vi "my_solution.vi"() -> ()   [LabVIEW 2013]
doc: "This example performs writes and reads on a serial port, as directed by the user. You can press the Write and Read buttons, and change the Read Count, while the example is running.\n\nThe parameters set for the serial port must match the parameters of the connected instrument or device. In this example, the Read Count parameter specifies the number of bytes that the serial port reads. If there were more bytes at the port than the specified number, those bytes would not be read. If there were less bytes at the port than the specified number, you would receive a timeout error.\n\nThis example expands upon the flow control options for XON and XOFF, allowing the user to choose those control characters. Also, the user can enable or disable a termination character. Some devices require a termination character in order to identify the end of command strings. Some devices send a termination character to signify the end of data to be read. This example shows how you can end the Read operation once a termination character is detected in the buffer and/or append a termination character at the end of the Write data."
uses:
  Program Files/National Instruments/LabVIEW 2013/examples/Instrument IO/Serial/support/Serial - Settings.ctl
  <vilib>/Instr/_visa.llb/VISA Configure Serial Port (Instr).vi
panel:
  out "device 4":bool
  out "device 3":bool
  out "Waveform Chart 9":T1(graph)
  out "Waveform Chart 8":T1(graph)
  out "Waveform Chart 7":T1(graph)
  out "unit type 3":dbl
  out "time3":dbl
  in  "Write 4":bool
  in  "Write 3":bool
  out "goniometer":u8(knob) scale=0.0..255.0
  out "unit type":dbl
  out "Waveform Chart 6":T1(graph)
  out "Waveform Chart 5":T1(graph)
  out "Waveform Chart 4":T1(graph)
  out "unit type 2":dbl
  out "time 2":dbl
  out "device 2":bool
  out "device 1":bool
  out "time":dbl
  in  "Write 2":bool
  out "Waveform Chart 3":T1(graph)
  out "Waveform Chart 2":T1(graph)
  out "Waveform Chart":T1(graph)
  in  "Stop":bool
  in  "Command":string="*IDN?"
  in  "Write":bool
  in  "Serial Settings":T2={"baud rate"=115200, "data bits"=8, "parity"=enum."None", "stop bits"=10, "flow control"=0} {"flow control" items=["None"=0, "XON/XOFF"=1, "RTS/CTS"=2, "DTR/DSR"=4]; "stop bits" items=["1.0"=10, "1.5"=15, "2.0"=20]; "data bits" min=5 max=8 step=1; "baud rate" items=["75"=75, "110"=110, "134"=134, "150"=150, "300"=300, "600"=600, "1200"=1200, "1800"=1800, "2400"=2400, "4800"=4800, "7200"=7200, "9600"=9600, "14400"=14400, "19200"=19200, "28800"=28800, "38400"=38400, "56000"=56000, "57600"=57600, "115200"=115200, "128000"=128000, "230400"=230400]}
  in  "VISA resource name":refnum<visa-resource-name>="COM4"
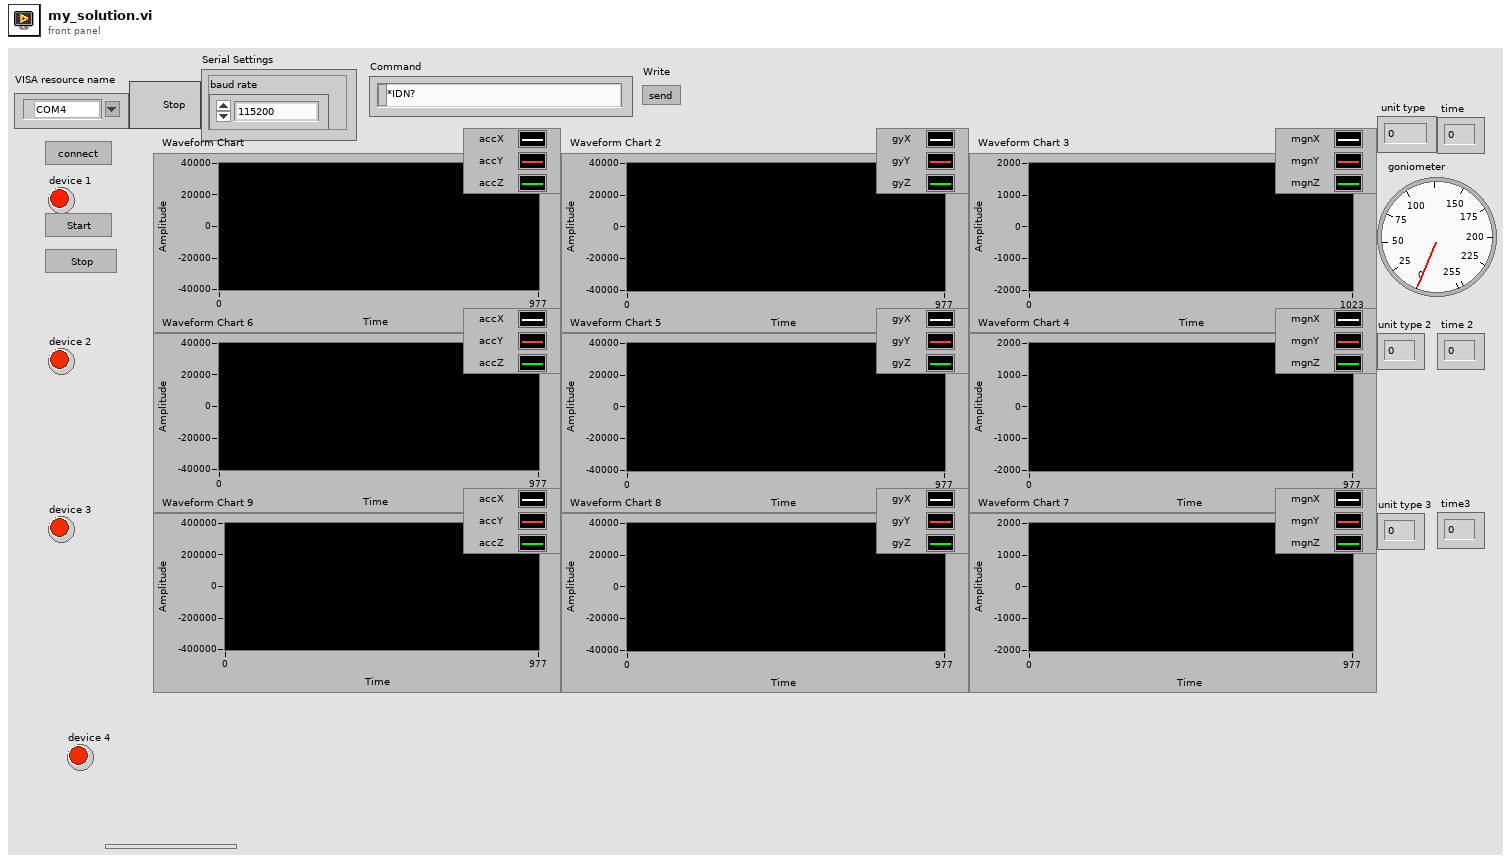
[diagram p1: front panel]
types:
  T1 = cluster{"Numeric Control":dbl, "Numeric Control":dbl, "Numeric Control":dbl}
  T2 = typedef "Serial - Settings.ctl" = cluster{"baud rate":u32, "data bits":u16, "parity":enum16{"None", "Odd", "Even", "Mark", "Space"}, "stop bits":u16, "flow control":u16}
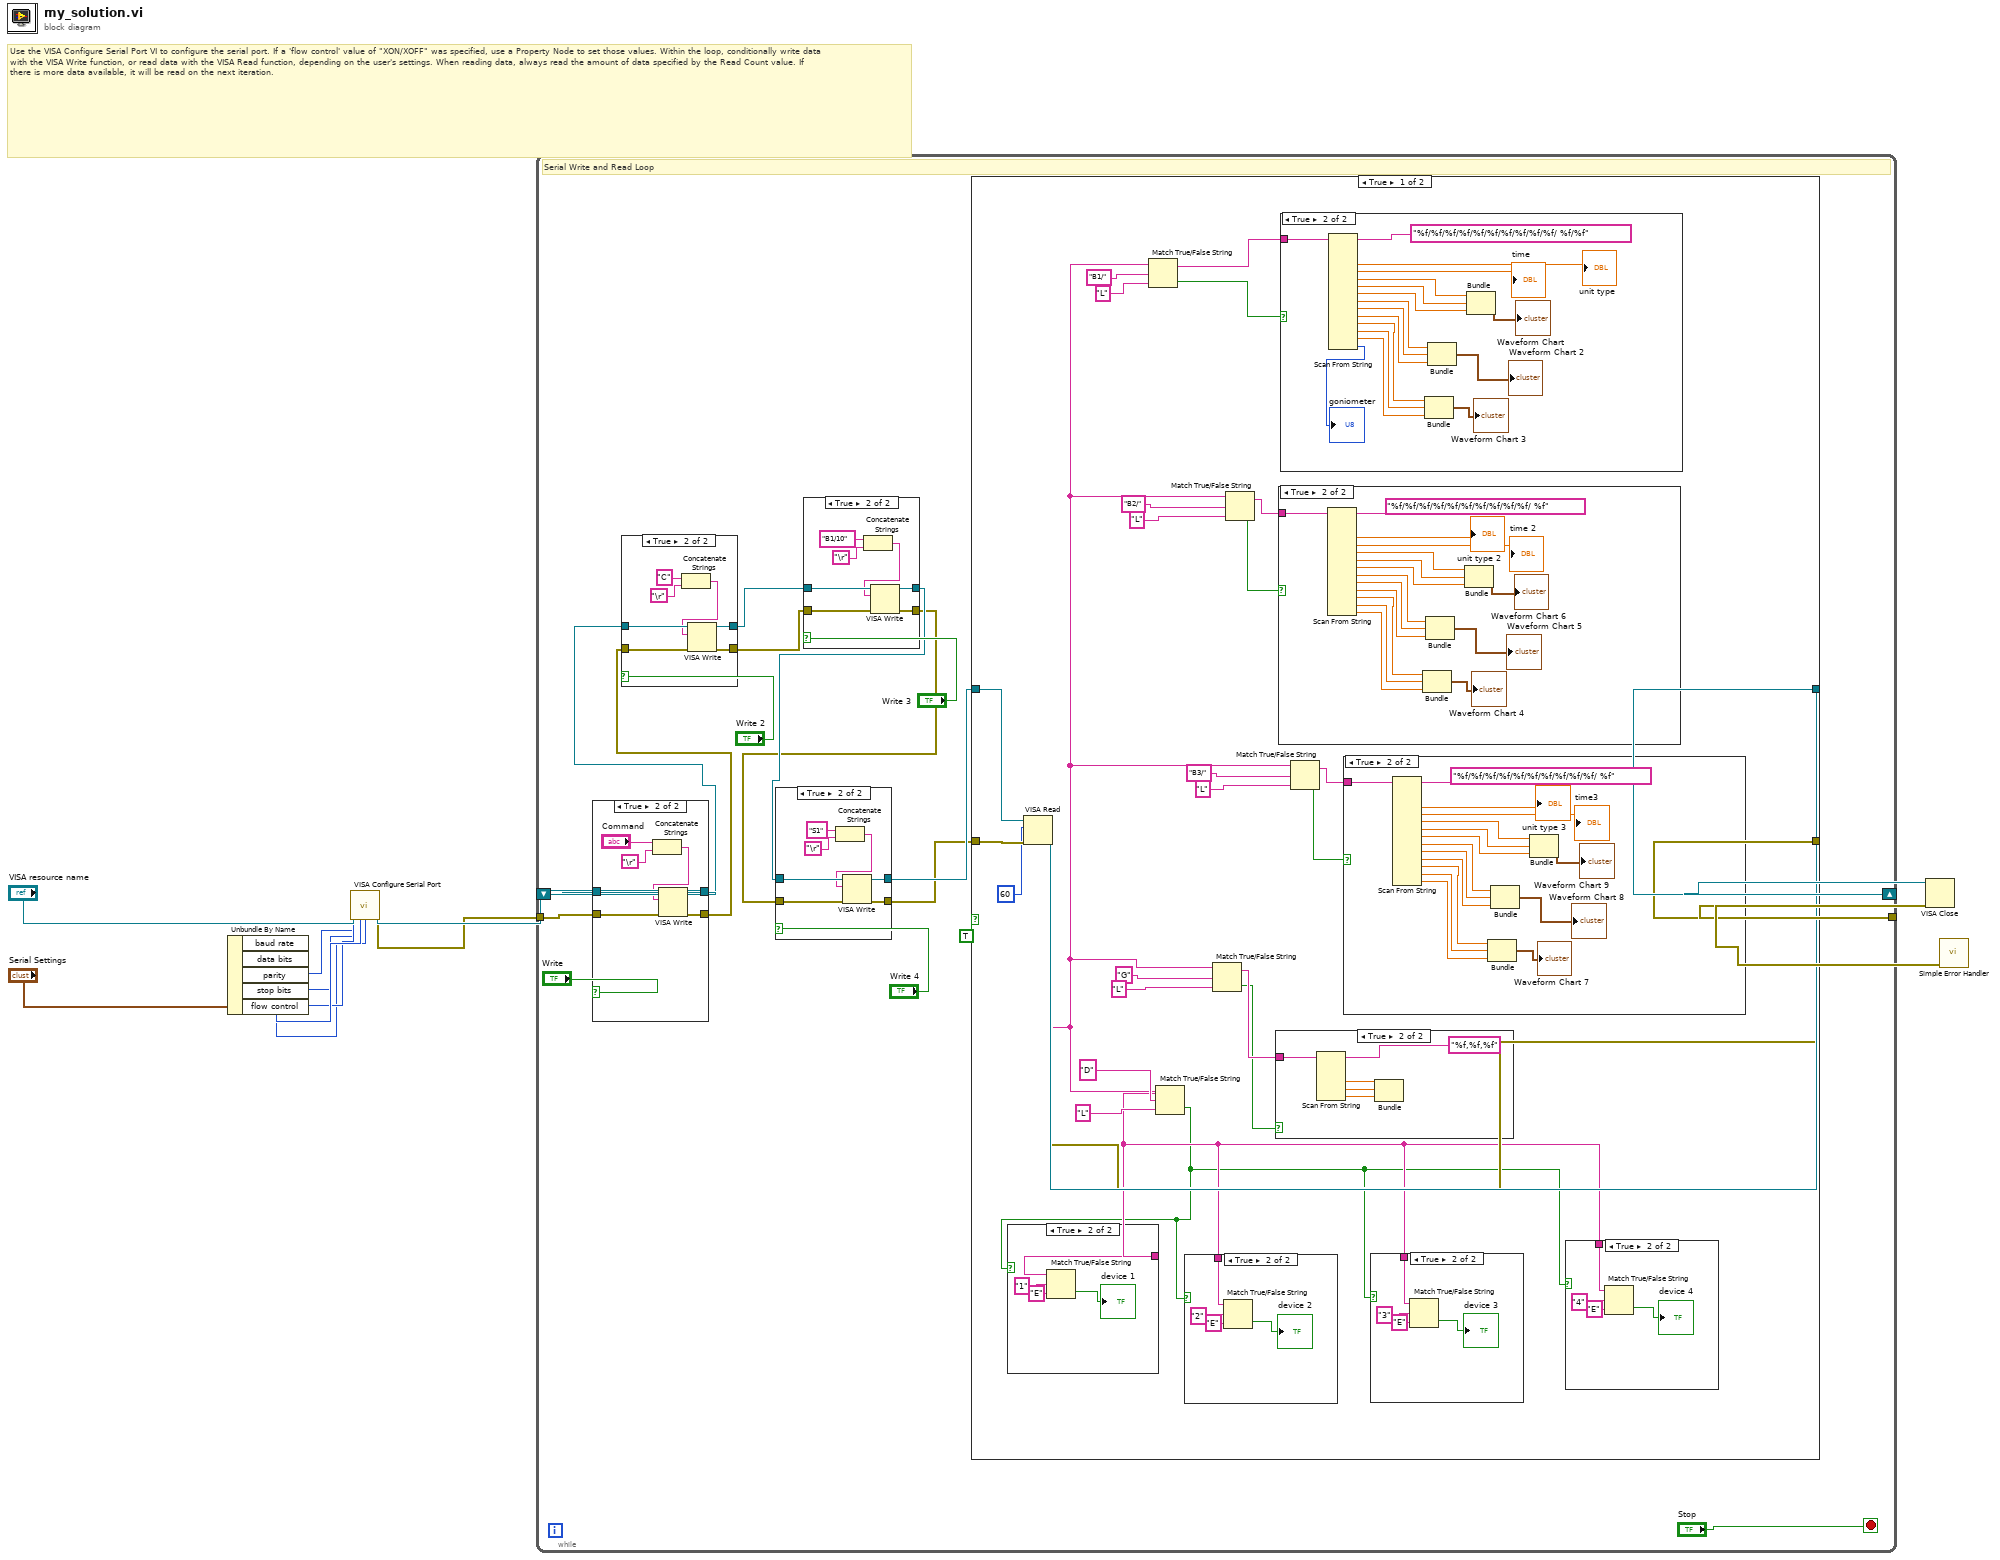
[diagram p0: block diagram]
diagram:
  # "Use the VISA Configure Serial Port VI to configure the serial port. If a 'flow control' value of \"XON/XOFF\" was specified, use a Property Node to set those values. Within the loop, conditionally write data with the VISA Write function, or read data with the VISA Read function, depending on the user's settings. When reading data, always read the amount of data specified by the Read Count value. If there is more data available, it will be read on the next iteration."
  n1 = Unbundle By Name("Serial Settings") -> ("baud rate"=w8:u32, "data bits"=w9:u16, "parity"=w10:enum16{"None", "Odd", "Even", "Mark", "Space"}, "stop bits"=w11:u16, "flow control"=w3:u16)
  n2 = call-poly "VISA Configure Serial Port"("VISA resource name"="VISA resource name", "baud rate (9600)"=w8, "data bits (8)"=w9, "parity (0:none)"=w10, "stop bits (10: 1 bit)"=w11, "flow control (0:none)"=w3) -> ("VISA resource name out"=w2:refnum<visa-resource-name>, "error out"=w1:errorcluster)  [unwired: 4 in, 4 out]
  n3 = while {
    shift-right: [w30] -> w4
    shift-left: w2 -> [w29]
    tunnel: w1 -> [w28]
    tunnel: [w27] -> w5
    stop <- "Stop" stop-if-true
    # "Serial Write and Read Loop"
    n4 = case shown="True" "Write" {
      tunnel: w29 -> [w59 w66]
      tunnel: w28 -> [w58 w65]
      tunnel: [w59 w64] -> w23
      tunnel: [w58 w63] -> w18
      frame False {
      }
      frame True {
        n5 = Concatenate Strings("Command", "\r") -> (w61:string)
        n6 = VISA Write(VISA resource name=w66, write buffer=w61, error in (no error)=w65) -> (VISA resource name out=w64:refnum<visa-resource-name>, error out=w63:errorcluster)  [unwired: 1 out]
      }
    }
    n7 = case shown="True" "Write 2" {
      tunnel: w23 -> [w50 w57]
      tunnel: w18 -> [w49 w52]
      tunnel: [w50 w56] -> w20
      tunnel: [w49 w55] -> w19
      frame False {
      }
      frame True {
        n8 = Concatenate Strings("C" ("string"), "\r") -> (w54:string)
        n9 = VISA Write(VISA resource name=w57, write buffer=w54, error in (no error)=w52) -> (VISA resource name out=w56:refnum<visa-resource-name>, error out=w55:errorcluster)  [unwired: 1 out]
      }
    }
    n10 = case shown="True" "Write 3" {
      tunnel: w20 -> [w41 w48]
      tunnel: w19 -> [w40 w43]
      tunnel: [w41 w47] -> w16
      tunnel: [w40 w46] -> w15
      frame False {
      }
      frame True {
        n11 = Concatenate Strings("B1/10" ("string"), "\r") -> (w45:string)
        n12 = VISA Write(VISA resource name=w48, write buffer=w45, error in (no error)=w43) -> (VISA resource name out=w47:refnum<visa-resource-name>, error out=w46:errorcluster)  [unwired: 1 out]
      }
    }
    n13 = case shown="True" "Write 4" {
      tunnel: w16 -> [w32 w39]
      tunnel: w15 -> [w31 w34]
      tunnel: [w32 w38] -> w14
      tunnel: [w31 w37] -> w13
      frame False {
      }
      frame True {
        n14 = Concatenate Strings("S1" ("string"), "\r") -> (w36:string)
        n15 = VISA Write(VISA resource name=w39, write buffer=w36, error in (no error)=w34) -> (VISA resource name out=w38:refnum<visa-resource-name>, error out=w37:errorcluster)  [unwired: 1 out]
      }
    }
    n16 = case shown="True" TRUE {
      tunnel: [w90 w164] -> w30
      tunnel: w14 -> [w92 w164]
      tunnel: [w87 w163] -> w27
      tunnel: w13 -> [w91 w163]
      frame True {
        n17 = VISA Read(VISA resource name=w92, byte count=u32 60, error in (no error)=w91) -> (VISA resource name out=w90:refnum<visa-resource-name>, read buffer=w69:string, error out=w87:errorcluster)  [unwired: 1 out]
        n18 = Match True/False String(2:"L" ("false string"), 3:"B1/" ("true string"), 4:w69) -> (0:w79:bool, 1:w80:string)
        n19 = Match True/False String(2:"L" ("false string"), 3:"D" ("true string"), 4:w69) -> (0:w67:bool, 1:w68:string)
        n20 = case shown="True" w67 {
          tunnel: w68 -> [_ w157]
          frame False {
          }
          frame True {
            n21 = Match True/False String(2:"E" ("false string"), 3:"1" ("true string"), 4:w157) -> (0:→"device 1":bool)  [unwired: 1 out]
          }
        }
        n22 = case shown="True" w67 {
          tunnel: w68 -> [_ w151]
          frame False {
          }
          frame True {
            n23 = Match True/False String(2:"E" ("false string"), 3:"2" ("true string"), 4:w151) -> (0:→"device 2":bool)  [unwired: 1 out]
          }
        }
        n24 = Match True/False String(2:"L" ("false string"), 3:"G" ("true string"), 4:w69) -> (0:w81:bool, 1:w82:string)
        n25 = Match True/False String(2:"L" ("false string"), 3:"B2/" ("true string"), 4:w69) -> (0:w75:bool, 1:w76:string)
        n26 = case shown="True" w81 {
          tunnel: w82 -> [_ w158]
          frame False {
          }
          frame True {
            n27 = Scan From String(format string="%f,%f,%f", input string=w158) -> (output 1=w161:dbl, output 2=w160:dbl, output 3=w159:dbl)  [unwired: 5 in, 3 out]
            n28 = Bundle(w161, w160, w159) -> ()  [unwired: 1 in, 1 out]
          }
        }
        n29 = case shown="True" w75 {
          tunnel: w76 -> [_ w146]
          frame False {
          }
          frame True {
            n30 = Scan From String(format string="%f/%f/%f/%f/%f/%f/%f/%f/%f/%f/ %f", input string=w146) -> (output 1=→"unit type 2":dbl, output 2=→"time 2":dbl, output 3=w145:dbl, output 4=w144:dbl, output 5=w143:dbl, output 6=w142:dbl, output 7=w141:dbl, output 8=w140:dbl, output 9=w138:dbl, output 10=w137:dbl, output 11=w136:dbl)  [unwired: 13 in, 3 out]
            n31 = Bundle(w138, w137, w136) -> (→"Waveform Chart 4":cluster{dbl, dbl, dbl})  [unwired: 1 in]
            n32 = Bundle(w142, w141, w140) -> (→"Waveform Chart 5":cluster{dbl, dbl, dbl})  [unwired: 1 in]
            n33 = Bundle(w145, w144, w143) -> (→"Waveform Chart 6":cluster{dbl, dbl, dbl})  [unwired: 1 in]
          }
        }
        n34 = case shown="True" w79 {
          tunnel: w80 -> [_ w119]
          frame False {
          }
          frame True {
            n35 = Scan From String(format string="%f/%f/%f/%f/%f/%f/%f/%f/%f/%f/ %f/%f", input string=w119) -> (output 1=→"unit type":dbl, output 2=→"time":dbl, output 3=w130:dbl, output 4=w129:dbl, output 5=w128:dbl, output 6=w127:dbl, output 7=w126:dbl, output 8=w125:dbl, output 9=w123:dbl, output 10=w122:dbl, output 11=w121:dbl, output 12=→"goniometer":u8)  [unwired: 14 in, 3 out]
            n36 = Bundle(w123, w122, w121) -> (→"Waveform Chart 3":cluster{dbl, dbl, dbl})  [unwired: 1 in]
            n37 = Bundle(w127, w126, w125) -> (→"Waveform Chart 2":cluster{dbl, dbl, dbl})  [unwired: 1 in]
            n38 = Bundle(w130, w129, w128) -> (→"Waveform Chart":cluster{dbl, dbl, dbl})  [unwired: 1 in]
          }
        }
        n39 = Match True/False String(2:"L" ("false string"), 3:"B3/" ("true string"), 4:w69) -> (0:w70:bool, 1:w71:string)
        n40 = case shown="True" w70 {
          tunnel: w71 -> [_ w113]
          frame False {
          }
          frame True {
            n41 = Scan From String(format string="%f/%f/%f/%f/%f/%f/%f/%f/%f/%f/ %f", input string=w113) -> (output 1=→"unit type 3":dbl, output 2=→"time3":dbl, output 3=w112:dbl, output 4=w111:dbl, output 5=w110:dbl, output 6=w109:dbl, output 7=w108:dbl, output 8=w107:dbl, output 9=w105:dbl, output 10=w104:dbl, output 11=w103:dbl)  [unwired: 13 in, 3 out]
            n42 = Bundle(w105, w104, w103) -> (→"Waveform Chart 7":cluster{dbl, dbl, dbl})  [unwired: 1 in]
            n43 = Bundle(w109, w108, w107) -> (→"Waveform Chart 8":cluster{dbl, dbl, dbl})  [unwired: 1 in]
            n44 = Bundle(w112, w111, w110) -> (→"Waveform Chart 9":cluster{dbl, dbl, dbl})  [unwired: 1 in]
          }
        }
        n45 = case shown="True" w67 {
          tunnel: w68 -> [_ w98]
          frame False {
          }
          frame True {
            n46 = Match True/False String(2:"E" ("false string"), 3:"3" ("true string"), 4:w98) -> (0:→"device 3":bool)  [unwired: 1 out]
          }
        }
        n47 = case shown="True" w67 {
          tunnel: w68 -> [_ w94]
          frame False {
          }
          frame True {
            n48 = Match True/False String(2:"E" ("false string"), 3:"4" ("true string"), 4:w94) -> (0:→"device 4":bool)  [unwired: 1 out]
          }
        }
      }
      frame False {
      }
    }
  }
  n49 = VISA Close(VISA resource name=w4, error in (no error)=w5) -> (error out=w6:errorcluster)
  n50 = call <vilib>:"Simple Error Handler.vi"("error in (no error)"=w6) -> ()  [unwired: 1 in, 8 out]
